vi "DeviceControl.vi"(11 "stop":refnum<vi>) -> (3 "status":string="running")   [LabVIEW 2013]
uses:
  Controls/diagnosticQuee.ctl
  Shared/MySQL/Preset Query Enum.ctl
  Controls/comunicationQueuecluster.ctl
  Controls/stopQue.ctl
  Controls/PingQueueTypDef.ctl
  Controls/deviceQueue.ctl
panel:
  out "error history":string[](array[string])
  in  "Device selected":bool[](array[boolean])=[FALSE, FALSE, FALSE, FALSE, FALSE, FALSE, FALSE, FALSE, FALSE, FALSE, FALSE, FALSE, FALSE, FALSE, FALSE, FALSE, FALSE, FALSE, FALSE, FALSE, FALSE, FALSE, FALSE, FALSE, FALSE, FALSE, FALSE, FALSE, FALSE, FALSE, FALSE, FALSE, FALSE, FALSE, FALSE, FALSE, FALSE, FALSE, FALSE, FALSE, FALSE, FALSE, FALSE, FALSE, FALSE, FALSE, FALSE, FALSE, FALSE, FALSE, FALSE, FALSE, FALSE, FALSE, FALSE, FALSE, FALSE, FALSE, FALSE, FALSE, FALSE, FALSE, FALSE, FALSE, FALSE, FALSE, FALSE, FALSE, FALSE, FALSE, FALSE, FALSE, FALSE, FALSE, FALSE, FALSE, FALSE, FALSE, FALSE, FALSE, FALSE, FALSE, FALSE, FALSE, FALSE, FALSE, FALSE, FALSE, FALSE, FALSE, FALSE, FALSE, FALSE, FALSE, FALSE, FALSE, FALSE, FALSE, FALSE]
  in  "error selected":bool[](array[boolean])=[TRUE, TRUE, TRUE, FALSE, TRUE, TRUE, TRUE, TRUE, TRUE, TRUE, TRUE, TRUE, TRUE, TRUE, TRUE, TRUE, TRUE, FALSE, FALSE, TRUE, FALSE, TRUE, TRUE, TRUE, FALSE, FALSE, TRUE, FALSE, TRUE, TRUE, FALSE, TRUE, TRUE, FALSE, FALSE, TRUE, FALSE, TRUE, FALSE, FALSE, TRUE, TRUE, FALSE]
  out "ststus":string[](array[string])=["Initialized", "Initialized", "Initialized", "Initialized", "Initialized", "Initialized", "Initialized", "Initialized", "Initialized", "Initialized", "Initialized", "Initialized", "Initialized", "Initialized", "Initialized", "Initialized", "Initialized", "Initialized", "Initialized", "Initialized", "Initialized", "Initialized", "Initialized", "Initialized", "Initialized", "Initialized", "Initialized", "Initialized", "Initialized", "Initialized", "Initialized", "Initialized", "Initialized", "Initialized", "Initialized", "Initialized", "Initialized", "Initialized", "Initialized", "Initialized", "Initialized", "Initialized", "Initialized"]
  out "error":string[](array[string])=["no error", "no error", "no error", "error", "no error", "no error", "no error", "no error", "no error", "no error", "no error", "no error", "no error", "no error", "no error", "no error", "no error", "error", "error", "no error", "error", "no error", "no error", "no error", "error", "error", "no error", "error", "no error", "no error", "error", "no error", "no error", "error", "error", "no error", "error", "no error", "error", "error", "no error", "no error", "error"]
  out "device":string[](array[string])=["StagingM1Far", "StagingM1Near", "StagingM3Far", "StagingM5", "StagingOAP2Near", "StagingOAP1Near", "StagingPXISlow", "StagingOAP2Far", "StagingLowPressure1", "StagingHexapodPI", "StagingDG645_1", "StagingLowPressure2", "StagingPXIFast2", "StagingPXIFast1", "StagingAlignBeam1", "StagingAlignBeam2", "StagingFilterWheels", "StagingShotControl", "StagingDG645_2", "StagingTRA3", "StagingGuppy", "TREX PXI fast", "StagingNISwitch", "StagingEnergy", "StagingTelescopePosition", "StagingDischargePower", "StagingDischargeHV", "StagingInterlock", "StagingAnalysisSlow", "Staging1Wire", "StagingTRA2", "StagingTelescopeImageLocation", "StagingBeam1OAPMotors", "StagingM4", "StagingDelayStage", "StagingTRA1", "StagingOAP1Far", "StagingFocusPositionBeam1", "StagingFocusPositionBeam2", "TREX TRA1", "StagingHighPressureDAQ", "StagingHighPressureController", "StagingTiming"]
  out "XY Graph":cluster{u32[], "Ramp Pattern":dbl[]}(graph)={[880, 160, 104, 38, 200, 39, 106, 65, 141, 118, 27, 317, 41, 159, 47, 61, 44, 165, 319, 58, 77, 430, 73, 122, 108, 55, 101, 70, 82, 884, 579, 178, 0, 114, 137, 100, 256, 83, 72, 157, 115, 129, 37], "Ramp Pattern"=[0.0, 1.0, 2.0, 3.0, 4.0, 5.0, 6.0, 7.0, 8.0, 9.0, 10.0, 11.0, 12.0, 13.0, 14.0, 15.0, 16.0, 17.0, 18.0, 19.0, 20.0, 21.0, 22.0, 23.0, 24.0, 25.0, 26.0, 27.0, 28.0, 29.0, 30.0, 31.0, 32.0, 33.0, 34.0, 35.0, 36.0, 37.0, 38.0, 39.0, 40.0, 41.0, 42.0]}
  in  "Stop":bool=TRUE
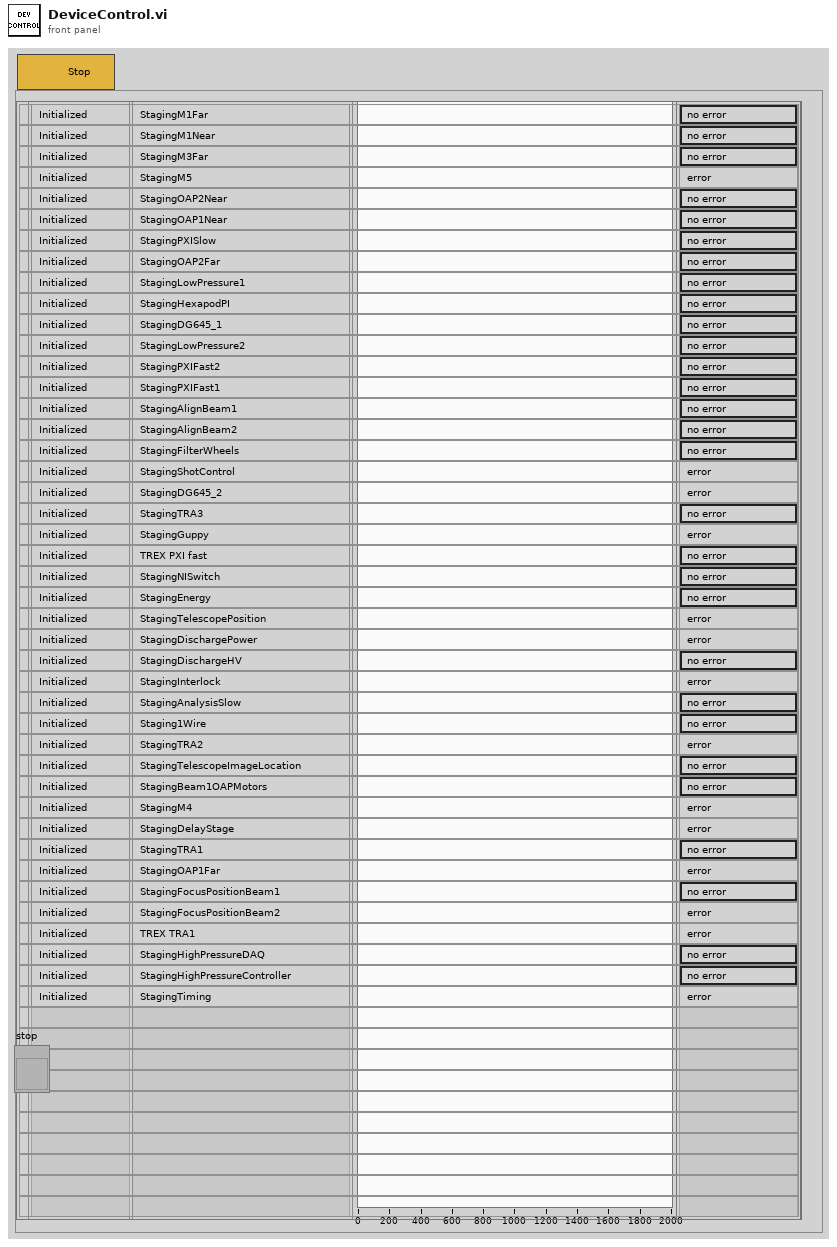
[diagram p1: front panel]
types:
  T1 = typedef "deviceQueue.ctl" = cluster{"device":string[], "XY Graph":cluster{"x":u32[], "Ramp Pattern":dbl[]}, "ststus":string[], "error":string[], "error history":string[]}
  T2 = typedef "PingQueueTypDef.ctl" = cluster{"Computers not on":string[]}
  T3 = typedef "stopQue.ctl" = cluster{"stop":bool}
  T4 = typedef "comunicationQueuecluster.ctl" = cluster{"device":string, "error history":string, "stop":bool}
  T5 = typedef "Preset Query Enum.ctl" = enum16{"Get Locations", "Get all IPs and MACs", "Get classes", "Get expt variables to set at scanstart for particular device", "Get expt devices and variables with start values", "Get expt devices and variables (with data to get)", "Get expt devices with data to get", "Get Expt devices and GUIs", "Get all devices basic properties", "Get Virtual Devices Core Info", "Get Expt names", "Get experiment basic properties", "Get experiment alarm variables", "Get MC Ports", "Get device network comm port", "Get devicetype lvclass path", "Get basic device properties", "Get Init Order", "Get all setable variables of a device", "Get device variable aliases", "Get force values of all settable variables", "Get all variables of a devicetype", "Get all variables of a device", "Get plotter details", "Get Saved Scans", "Get Scan Info", "GetGeneralGUIs", "Get expt for plotter", "Get plotter IDs from expt", "Get all devices", "Get all Virtual Devices", "Get all aliases", "Get variable and device info for Virtual Device", "GetItemLocatorIP", "Get IPs for GUIs", "Get DeviceType from Device", "GetLocalPortRange", "GetDevicePresetVariables", "Get Device Configuration", "GetAllPresetNames", "GetAllConfigurationNames", "GetPresetDeviceNames"}
  T6 = typedef "diagnosticQuee.ctl" = cluster{"device":string[], "error":string[], "ststus":string[], "timing graph":cluster{u32[], "Ramp Pattern":dbl[]}, "error boolean":bool[], "error history":string[]}
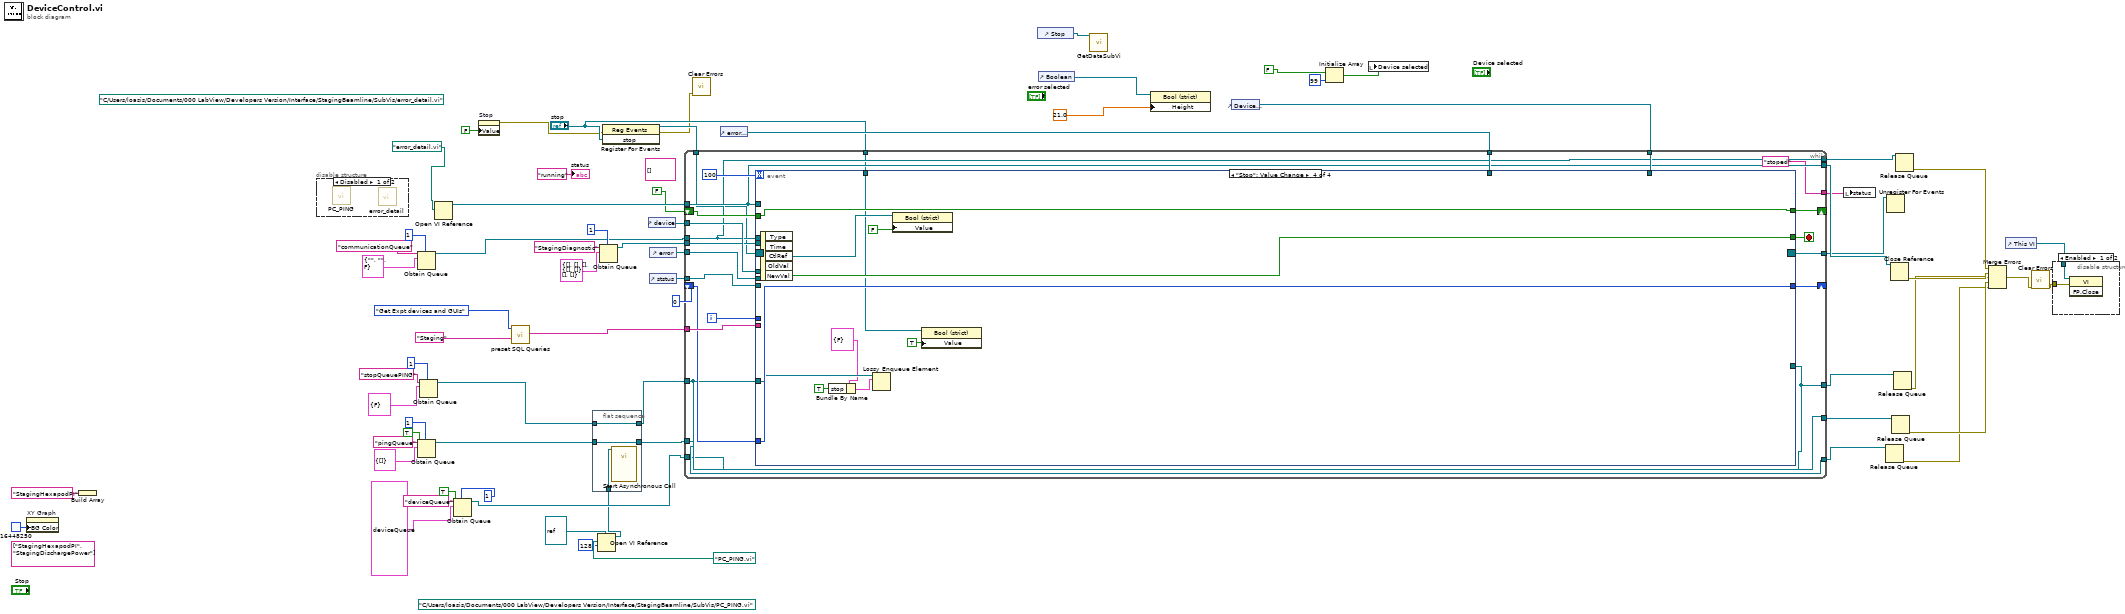
[diagram p0: block diagram]
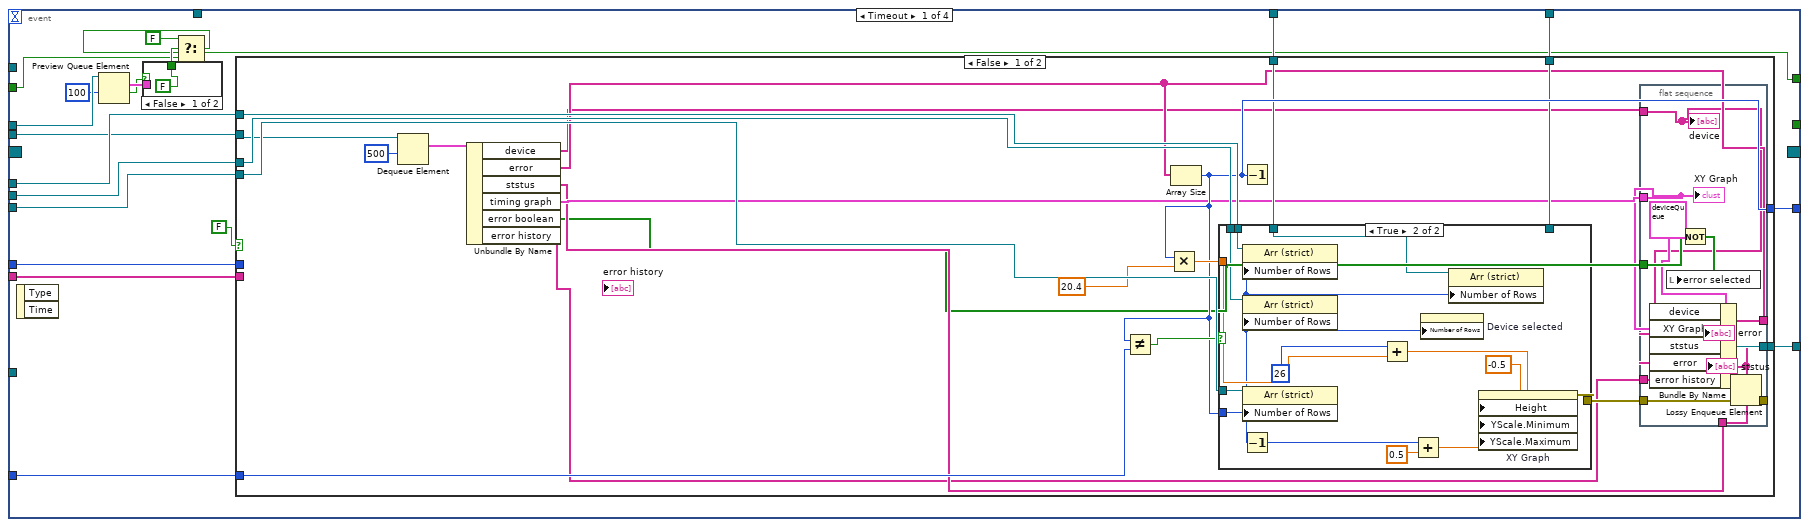
[diagram p4: hidden frame]
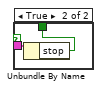
[diagram p5: hidden frame]
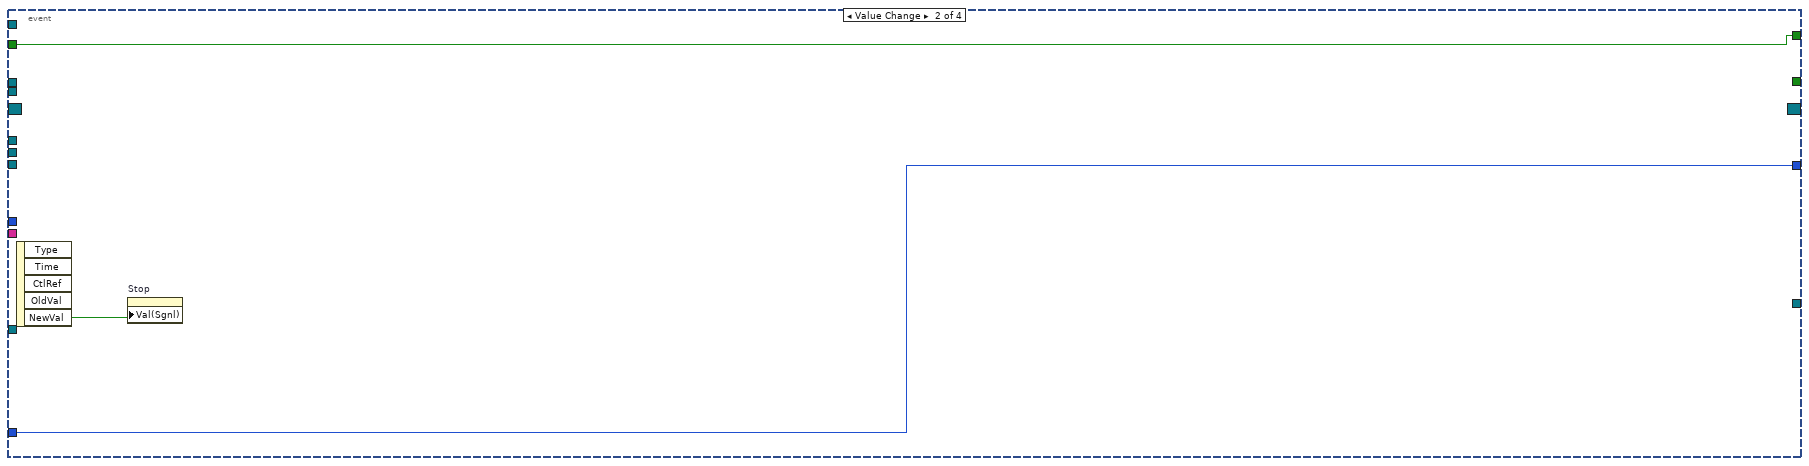
[diagram p8: hidden frame]
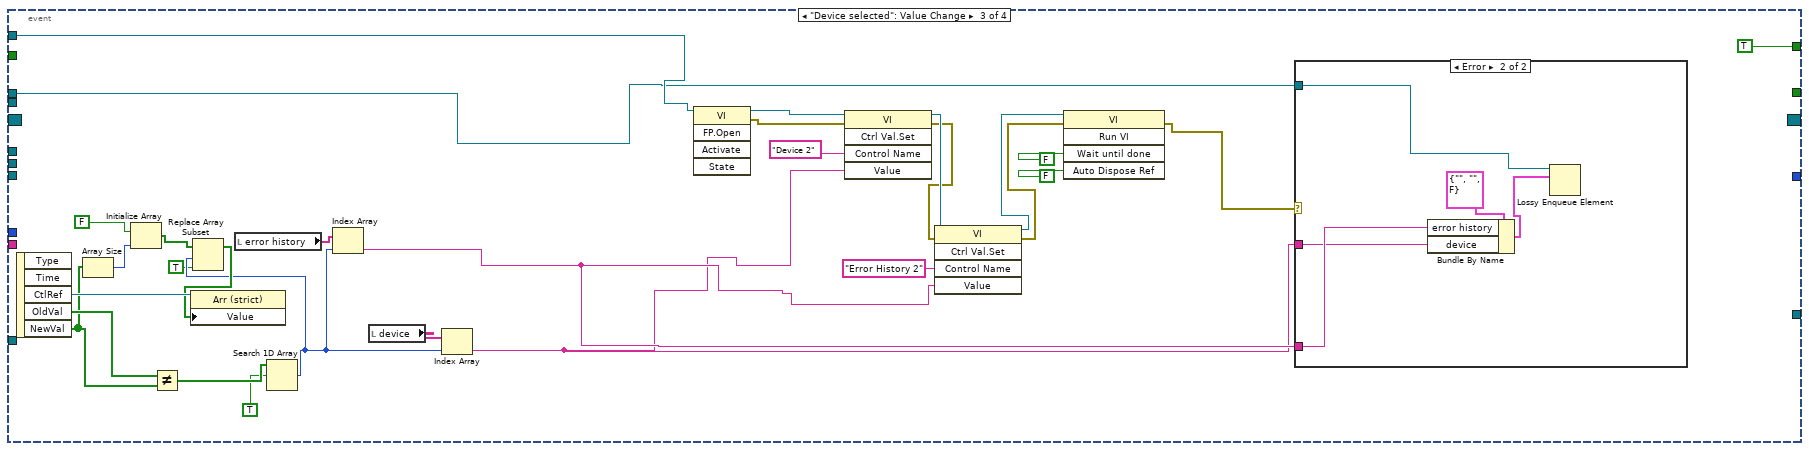
[diagram p9: hidden frame]
diagram:
  (unwired) path "C:/Users/loasis/Documents/000 LabView/Developers Version/Interface/StagingBeamline/SubVis/PC_PING.vi" ("vi path")
  (unwired) path "C:/Users/loasis/Documents/000 LabView/Developers Version/Interface/StagingBeamline/SubVis/error_detail.vi" ("vi path")
  (unwired) string[][] []
  (unwired) string[] ["StagingHexapodPI", "StagingDischargePower"]
  n1 = property on="XY Graph" class="XYGraph (strict)"("BG Color"=u32 16448250) -> ()  [unwired: 2 in, 2 out]
  n2 = Build Array("StagingHexapodPI" ("String")) -> ()  [unwired: 1 out]
  n3 = disable-structure shown="Disabled" {
    frame Disabled {
      n4 = call "PC_PING.vi"() -> ()  [unwired: 12 in]
      n5 = call "error_detail.vi"() -> ()  [unwired: 12 in]
    }
    frame Enabled {
    }
  }
  n6 = Obtain Queue(max queue size (-1, unlimited)=1, name (unnamed)="communicationQueue", element data type=T4 {"device"="", "error history"="", "stop"=FALSE}) -> (queue out=w42:refnum<queue>)  [unwired: 2 in, 2 out]
  n7 = Obtain Queue(max queue size (-1, unlimited)=1, name (unnamed)="pingQueue", element data type=T2 {"Computers not on"=[]}, create if not found? (T)=TRUE) -> (queue out=w25:refnum<queue>)  [unwired: 1 in, 2 out]
  n8 = Obtain Queue(max queue size (-1, unlimited)=1, name (unnamed)="stopQueuePING", element data type=T3 {"stop"=FALSE}) -> (queue out=w23:refnum<queue>)  [unwired: 2 in, 2 out]
  n9 = Open VI Reference(vi path=path "error_detail.vi") -> (vi reference=w47:refnum<vi>)  [unwired: 5 in, 1 out]
  n10 = Obtain Queue(max queue size (-1, unlimited)=1, name (unnamed)="deviceQueue", element data type=T1 {"device"=["StagingM1Far", "StagingM1Near", "StagingM3Far", "StagingM5", "StagingOAP2Near", "StagingOAP1Near", "StagingPXISlow", "StagingOAP2Far", "StagingLowPressure1", "StagingHexapodPI", "StagingDG645_1", "StagingLowPressure2", "StagingPXIFast2", "StagingPXIFast1", "StagingAlignBeam1", "StagingAlignBeam2", "StagingFilterWheels", "StagingShotControl", "StagingDG645_2", "StagingTRA3", "StagingGuppy", "TREX PXI fast", "StagingNISwitch", "StagingEnergy", "StagingTelescopePosition", "StagingDischargePower", "StagingDischargeHV", "StagingInterlock", "StagingAnalysisSlow", "Staging1Wire", "StagingTRA2", "StagingTelescopeImageLocation", "StagingBeam1OAPMotors", "StagingM4", "StagingDelayStage", "StagingTRA1", "StagingOAP1Far", "StagingFocusPositionBeam1", "StagingFocusPositionBeam2", "TREX TRA1", "StagingHighPressureDAQ", "StagingHighPressureController"], "XY Graph"={"x"=[154, 10000, 41, 80, 72, 7, 151, 45, 108, 239, 223, 116, 0, 109, 143, 4, 112, 224, 106, 57, 89, 58, 39, 40, 414, 148, 167, 127, 199, 314, 183, 174, 107, 5, 104, 505, 42, 76, 44, 102, 3, 30], "Ramp Pattern"=[0.0, 1.0, 2.0, 3.0, 4.0, 5.0, 6.0, 7.0, 8.0, 9.0, 10.0, 11.0, 12.0, 13.0, 14.0, 15.0, 16.0, 17.0, 18.0, 19.0, 20.0, 21.0, 22.0, 23.0, 24.0, 25.0, 26.0, 27.0, 28.0, 29.0, 30.0, 31.0, 32.0, 33.0, 34.0, 35.0, 36.0, 37.0, 38.0, 39.0, 40.0, 41.0]}, "ststus"=["Initialized", "Initialized", "Initialized", "Initialized", "Initialized", "Initialized", "Initialized", "Initialized", "Initialized", "Initialized", "Initialized", "Initialized", "Initialized", "Initialized", "Initialized", "Initialized", "Initialized", "Initialized", "Initialized", "Initialized", "Initialized", "Initialized", "Initialized", "Initialized", "Initialized", "Initialized", "Initialized", "Initialized", "Initialized", "Initialized", "Initialized", "Initialized", "Initialized", "Initialized", "Initialized", "Initialized", "Initialized", "Initialized", "Initialized", "Initialized", "no response", "Initialized"], "error"=["no error", "no error", "no error", "error", "no error", "no error", "no error", "no error", "no error", "no error", "no error", "no error", "no error", "no error", "no error", "no error", "no error", "no error", "no error", "no error", "error", "no error", "no error", "no error", "no error", "no error", "no error", "no error", "no error", "no error", "no error", "no error", "no error", "no error", "no error", "no error", "no error", "no error", "no error", "no error", "no response", "no error"], "error history"=[]} ("deviceQueue"), create if not found? (T)=TRUE) -> (queue out=w27:refnum<queue>)  [unwired: 1 in, 2 out]
  n11 = property on="Stop" class="Bool (strict)"("Value"=FALSE) -> (error out=w1:errorcluster)  [unwired: 2 in, 1 out]
  n12 = call "preset SQL Queries.vi"("Expt name / MCIP/ Variable/Preset Name"="Staging" ("Expt name / MCIP/ Variable Name"), "Preset Query"=Preset_Query_Enum."Get Expt devices and GUIs") -> ("1st column 1st data"=w61:string[])  [unwired: 7 in, 2 out]
  n13 = flat-sequence {
    tunnel: w25 -> [w72]
    tunnel: [w72] -> w24
    tunnel: w23 -> [w71]
    tunnel: [w71] -> w22
    tunnel: w18 -> [w70]
    frame #0 {
      n14 = call-by-ref "Start Asynchronous Call"(reference=w70) -> ()  [unwired: 13 in, 2 out]
    }
  }
  n15 = Open VI Reference(type specifier VI Refnum (for type only)=refnum<vi> refnum, vi path=path "PC_PING.vi", options=128) -> (vi reference=w18:refnum<vi>)  [unwired: 3 in, 1 out]
  n16 = Obtain Queue(max queue size (-1, unlimited)=1, name (unnamed)="StagingDiagnostic", element data type=T6 {"device"=[], "error"=[], "ststus"=[], "timing graph"={[], "Ramp Pattern"=[]}, "error boolean"=[], "error history"=[]} ("output cluster")) -> (queue out=w50:refnum<queue>)  [unwired: 2 in, 2 out]
  n17 = register-events(error in=w1, "stop") -> (reference out=w8:refnum<event-registration>, error out=w2:errorcluster)  [unwired: 1 in]
  n18 = control-ref of="device"() -> (w65:refnum<vi>)
  n19 = control-ref of="error"() -> (w64:refnum<vi>)
  n20 = control-ref of="ststus"() -> (w66:refnum<vi>)
  n21 = call <vilib>:"Clear Errors.vi"("error in (no error)"=w2) -> ()  [unwired: 6 in, 1 out]
  n22 = control-ref of="error selected"() -> (w62:refnum<vi>)
  n23 = control-ref of="Stop"() -> (w54:refnum<vi>)
  n24 = control-ref of="Boolean"() -> (w55:refnum<vi>)
  n25 = call "GetDataSubVi.vi"("Stop 2"=w54) -> ()  [unwired: 11 in]
  n26 = property class="Bool (strict)"(reference=w55, "Height"=21.0 ("Numeric")) -> ()  [unwired: 1 in, 2 out]
  n27 = control-ref of="Device selected"() -> (w60:refnum<vi>)
  n28 = while {
    tunnel: w61 -> [w92]
    tunnel: w66 -> [w91]
    tunnel: w65 -> [w90]
    tunnel: w64 -> [w89]
    shift-right: [w88] -> _
    shift-left: u32 0 ("Number of Rows") -> [w87]
    tunnel: w62 -> [w86]
    tunnel: w60 -> [w85]
    tunnel: w50 -> [w84]
    tunnel: w47 -> [w83]
    tunnel: [w83] -> w46
    shift-right: [w81] -> _
    shift-left: FALSE -> [w82]
    tunnel: w42 -> [w80]
    tunnel: [w80] -> w41
    tunnel: w22 -> [w79]
    tunnel: [w79] -> w37
    tunnel: w24 -> [w78]
    tunnel: [w78] -> w32
    tunnel: w27 -> [w77]
    tunnel: [w77] -> w26
    tunnel: w8 -> [w76]
    tunnel: [w75] -> w7
    tunnel: ["stoped"] -> w5
    tunnel: "stop" -> [w73]
    i -> [w93]
    stop <- w95 stop-if-true
    n29 = event shown="[3] \"Stop\": Value Change" {
      selector: w76 -> [_ _ _ _]
      dyn-events: [_ _ _ _] -> w75
      timeout: 100 -> [_ _ _ _]
      tunnel: [_ _ _ w212] -> w95
      tunnel: w93 -> [w115 _ _ _]
      tunnel: w92 -> [w107 _ _ _]
      tunnel: w91 -> [w114 _ _ _]
      tunnel: w90 -> [w113 _ _ _]
      tunnel: w89 -> [w112 _ _ _]
      tunnel: [w111 w167 _ w211] -> w88
      tunnel: w87 -> [w110 w167 _ w211]
      tunnel: w86 -> [w109 _ _ _]
      tunnel: w85 -> [w108 _ _ _]
      tunnel: w84 -> [w106 _ _ _]
      tunnel: w83 -> [_ _ w192 _]
      tunnel: w82 -> [w99 w166 _ w208]
      tunnel: [w100 w166 TRUE w208] -> w81
      tunnel: w80 -> [w103 _ w180 _]
      tunnel: w79 -> [_ _ _ w207]
      tunnel: w77 -> [w104 _ _ _]
      tunnel: w73 -> [_ _ _ w202]
      event Timeout {
        n30 = event-data() -> ()  [unwired: 1 in, 2 out]
        n31 = Preview Queue Element(queue=w103, timeout in ms (-1)=100) -> (element=w102:T4, timed out?=w96:bool)  [unwired: 1 in, 2 out]
        n32 = case shown="False" w96 {
          tunnel: w102 -> [_ w118]
          tunnel: [FALSE w117] -> w101
          frame False {
          }
          frame True {
            n33 = Unbundle By Name(w118) -> ("stop"=w117:bool)
          }
        }
        n34 = Select(t=FALSE, s=w101, f=w99) -> (s? t:f=w100:bool)
        n35 = case shown="False" FALSE {
          tunnel: w115 -> [_ _]
          tunnel: w107 -> [_ _]
          tunnel: w114 -> [w139 _]
          tunnel: w113 -> [w138 _]
          tunnel: w112 -> [w137 _]
          tunnel: [w131 w164] -> w111
          tunnel: w110 -> [w133 w164]
          tunnel: w109 -> [w130 _]
          tunnel: w108 -> [w129 _]
          tunnel: w106 -> [w128 _]
          tunnel: w104 -> [w120 _]
          frame False {
            n36 = Dequeue Element(queue=w128, timeout in ms (-1)=500) -> (element=w127:T6)  [unwired: 1 in, 3 out]
            n37 = Unbundle By Name(w127) -> ("device"=w122:string[], "error"=w123:string[], "ststus"=w125:string[], "timing graph"=w126:cluster{u32[], "Ramp Pattern":dbl[]}, "error boolean"=w124:bool[], "error history"=w119:string[])
            n38 = Array Size(array=w123) -> (size(s)=w131:i32)
            n39 = Not Equal?(x=w131, y=w133) -> (x != y?=w132:bool)
            n40 = Multiply(x=w131, y=20.4) -> (x*y=w134:dbl)
            n41 = case shown="True" w132 {
              tunnel: w139 -> [_ w152]
              tunnel: w138 -> [_ w151]
              tunnel: w137 -> [_ w150]
              tunnel: [_ w146] -> w135
              tunnel: w131 -> [_ w140]
              tunnel: w134 -> [_ w144]
              tunnel: w130 -> [_ w141]
              tunnel: w129 -> [_ _]
              frame False {
              }
              frame True {
                n42 = Decrement(x=w140) -> (x-1=w145:i32)
                n43 = property class="Arr (strict)"(reference=w151, "Number of Rows"=w140) -> ()  [unwired: 1 in, 2 out]
                n44 = property class="Arr (strict)"(reference=w150, "Number of Rows"=w140) -> ()  [unwired: 1 in, 2 out]
                n45 = property class="Arr (strict)"(reference=w152, "Number of Rows"=w140) -> ()  [unwired: 1 in, 2 out]
                n46 = Add(x=u32 26, y=w144) -> (x+y=w142:dbl)
                n47 = Add(x=w145, y=0.5) -> (x+y=w147:dbl)
                n48 = property on="Device selected" class="Arr (strict)"("Number of Rows"=w140) -> ()  [unwired: 2 in, 2 out]
                n49 = property class="Arr (strict)"(reference=w141, "Number of Rows"=w140) -> ()  [unwired: 1 in, 2 out]
                n50 = property on="XY Graph" class="XYGraph (strict)"("Height"=w142, "YScale.Minimum"=-0.5 ("Y Scale.Range:Minimum"), "YScale.Maximum"=w147) -> (error out=w146:errorcluster)  [unwired: 2 in, 1 out]
              }
            }
            n51 = Decrement(x=w131) -> ()  [unwired: 1 out]
            n52 = flat-sequence {
              tunnel: w126 -> [w157]
              tunnel: [w163] -> _
              tunnel: w135 -> [w163]
              tunnel: w125 -> [w156]
              tunnel: w124 -> [w162]
              tunnel: w123 -> [w155]
              tunnel: w122 -> [w158]
              tunnel: w120 -> [w160]
              tunnel: w119 -> [w153]
              frame #0 {
                n53 = Bundle By Name(cluster=T1 {"device"=["StagingM1Far", "StagingM1Near", "StagingM3Far", "StagingM5", "StagingOAP2Near", "StagingOAP1Near", "StagingPXISlow", "StagingOAP2Far", "StagingLowPressure1", "StagingHexapodPI", "StagingDG645_1", "StagingLowPressure2", "StagingPXIFast2", "StagingPXIFast1", "StagingAlignBeam1", "StagingAlignBeam2", "StagingFilterWheels", "StagingShotControl", "StagingDG645_2", "StagingTRA3", "StagingGuppy", "TREX PXI fast", "StagingNISwitch", "StagingEnergy", "StagingTelescopePosition", "StagingDischargePower", "StagingDischargeHV", "StagingInterlock", "StagingAnalysisSlow", "Staging1Wire", "StagingTRA2", "StagingTelescopeImageLocation", "StagingBeam1OAPMotors", "StagingM4", "StagingDelayStage", "StagingTRA1", "StagingOAP1Far", "StagingFocusPositionBeam1", "StagingFocusPositionBeam2", "TREX TRA1", "StagingHighPressureDAQ", "StagingHighPressureController"], "XY Graph"={"x"=[154, 10000, 41, 80, 72, 7, 151, 45, 108, 239, 223, 116, 0, 109, 143, 4, 112, 224, 106, 57, 89, 58, 39, 40, 414, 148, 167, 127, 199, 314, 183, 174, 107, 5, 104, 505, 42, 76, 44, 102, 3, 30], "Ramp Pattern"=[0.0, 1.0, 2.0, 3.0, 4.0, 5.0, 6.0, 7.0, 8.0, 9.0, 10.0, 11.0, 12.0, 13.0, 14.0, 15.0, 16.0, 17.0, 18.0, 19.0, 20.0, 21.0, 22.0, 23.0, 24.0, 25.0, 26.0, 27.0, 28.0, 29.0, 30.0, 31.0, 32.0, 33.0, 34.0, 35.0, 36.0, 37.0, 38.0, 39.0, 40.0, 41.0]}, "ststus"=["Initialized", "Initialized", "Initialized", "Initialized", "Initialized", "Initialized", "Initialized", "Initialized", "Initialized", "Initialized", "Initialized", "Initialized", "Initialized", "Initialized", "Initialized", "Initialized", "Initialized", "Initialized", "Initialized", "Initialized", "Initialized", "Initialized", "Initialized", "Initialized", "Initialized", "Initialized", "Initialized", "Initialized", "Initialized", "Initialized", "Initialized", "Initialized", "Initialized", "Initialized", "Initialized", "Initialized", "Initialized", "Initialized", "Initialized", "Initialized", "no response", "Initialized"], "error"=["no error", "no error", "no error", "error", "no error", "no error", "no error", "no error", "no error", "no error", "no error", "no error", "no error", "no error", "no error", "no error", "no error", "no error", "no error", "no error", "error", "no error", "no error", "no error", "no error", "no error", "no error", "no error", "no error", "no error", "no error", "no error", "no error", "no error", "no error", "no error", "no error", "no error", "no error", "no error", "no response", "no error"], "error history"=[]} ("deviceQueue"), "device"=w158, "XY Graph"=w157, "ststus"=w156, "error"=w155, "error history"=w153) -> (w154:T1)
                n54 = Not(x=w162) -> (.not. x?=w161:bool[])
                n55 = local write "error selected"(w161) -> ()
                n56 = Lossy Enqueue Element(queue=w160, element=w154) -> ()  [unwired: 1 in, 4 out]
                "XY Graph" <- w157
                "device" <- w158
                "error" <- w155
                "ststus" <- w156
              }
            }
          }
          frame True {
          }
        }
      }
      event Value Change {
        n57 = event-data() -> ("NewVal"=w165:bool)  [unwired: 1 in, 4 out]
        n58 = property on="Stop" class="Bool (strict)"("Val(Sgnl)"=w165) -> ()  [unwired: 2 in, 2 out]
      }
      event "Device selected": Value Change {
        n59 = event-data() -> ("CtlRef"=w190:refnum<vi>, "OldVal"=w188:bool[], "NewVal"=w187:bool[])  [unwired: 1 in, 2 out]
        n60 = Array Size(array=w187) -> (size(s)=w186:i32)
        n61 = Initialize Array(FALSE, w186) -> (w185:bool[])
        n62 = Not Equal?(x=w188, y=w187) -> (x != y?=w196:bool[])
        n63 = local read "error history"() -> (w193:string[])
        n64 = Search 1D Array(1D array=w196, element=TRUE) -> (index of element=w183:i32)  [unwired: 1 in]
        n65 = Replace Array Subset(array=w185, new element=TRUE ("new element/subarray"), index=w183) -> (w184:bool[])
        n66 = property class="Arr (strict)"(reference=w190, "Value"=w184) -> ()  [unwired: 1 in, 2 out]
        n67 = Index Array(array=w193, index=w183) -> (element=w179:string)
        n68 = local read "device"() -> (w194:string[])
        n69 = Index Array(array=w194, index=w183) -> (element=w178:string)
        n70 = invoke class="VI" method="FP.Open"(reference=w192) -> (reference out=w176:refnum<vi>, error out=w170:errorcluster)  [unwired: 4 in, 3 out]
        n71 = invoke class="VI" method="Ctrl Val.Set"(reference=w176, error in=w170, "Control Name"="Device 2", "Value"=w178) -> (reference out=w173:refnum<vi>, error out=w169:errorcluster)  [unwired: 1 in, 3 out]
        n72 = invoke class="VI" method="Ctrl Val.Set"(reference=w173, error in=w169, "Control Name"="Error History 2", "Value"=w179) -> (reference out=w172:refnum<vi>, error out=w168:errorcluster)  [unwired: 1 in, 3 out]
        n73 = invoke class="VI" method="Run VI"(reference=w172, error in=w168, "Wait until done"=FALSE ("Wait Until Done"), "Auto Dispose Ref"=FALSE ("Auto Dispose Reference")) -> (error out=w181:errorcluster)  [unwired: 1 in, 4 out]
        n74 = case shown="Error" w181 {
          tunnel: w180 -> [_ w199]
          tunnel: w179 -> [_ w198]
          tunnel: w178 -> [_ w197]
          frame No Error {
          }
          frame Error {
            n75 = Bundle By Name(cluster=T4 {"device"="", "error history"="", "stop"=FALSE}, "error history"=w198, "device"=w197) -> (w201:T4)
            n76 = Lossy Enqueue Element(queue=w199, element=w201) -> ()  [unwired: 1 in, 4 out]
          }
        }
      }
      event "Stop": Value Change {
        n77 = event-data() -> ("CtlRef"=w210:refnum<vi>, "NewVal"=w212:bool)  [unwired: 1 in, 3 out]
        n78 = Bundle By Name(cluster=T3 {"stop"=FALSE}, "stop"=TRUE) -> (w204:T3)
        n79 = Lossy Enqueue Element(queue=w207, element=w204) -> ()  [unwired: 1 in, 4 out]
        n80 = property class="Bool (strict)"(reference=w210, "Value"=FALSE) -> ()  [unwired: 1 in, 2 out]
        n81 = property class="Bool (strict)"(reference=w202, "Value"=TRUE) -> ()  [unwired: 1 in, 2 out]
      }
    }
  }
  n82 = Initialize Array(FALSE, 99 ("dimension size")) -> (w57:bool[])
  n83 = local write "Device selected"(w57) -> ()
  n84 = local write "status"(w5) -> ()
  n85 = Release Queue(queue=w32) -> (error out=w12:errorcluster)  [unwired: 2 in, 2 out]
  n86 = Unregister For Events(event registration refnum=w7) -> ()  [unwired: 1 in, 1 out]
  n87 = Close Reference(reference=w46) -> (error out=w15:errorcluster)  [unwired: 1 in]
  n88 = Release Queue(queue=w37) -> (error out=w13:errorcluster)  [unwired: 2 in, 2 out]
  n89 = Release Queue(queue=w26) -> (error out=w14:errorcluster)  [unwired: 2 in, 2 out]
  n90 = Release Queue(queue=w41) -> (error out=w16:errorcluster)  [unwired: 2 in, 2 out]
  n91 = Merge Errors(w16, w15, w14, w13, w12) -> (w11:errorcluster)
  n92 = control-ref of="This VI"() -> (w9:refnum<vi>)
  n93 = call <vilib>:"Clear Errors.vi"("error in (no error)"=w11) -> ("error out"=w10:errorcluster)  [unwired: 6 in]
  n94 = disable-structure shown="Enabled" {
    disable-tunnel: w10 -> [w214 _]
    disable-tunnel: w9 -> [w213 _]
    frame Enabled {
      n95 = invoke class="VI" method="FP.Close"(reference=w213, error in=w214) -> ()  [unwired: 1 in, 3 out]
    }
    frame Disabled {
    }
  }
  "status" <- "running"
